vi "CRYAPI DOCKING LIB.vi"(6 "sData":string, 8 "tDFrame":T2, 9 "tSFrame":T2, 10 "nData":i32=2, 11 "sAction":string) -> (0 "nData_Out":i32=2, 1 "sData_Out":string, 3 "tFrame_Out":T2)   [LabVIEW 2013]
uses:
  <vilib>/Utility/miscctls.llb/LVRectTypeDef.ctl
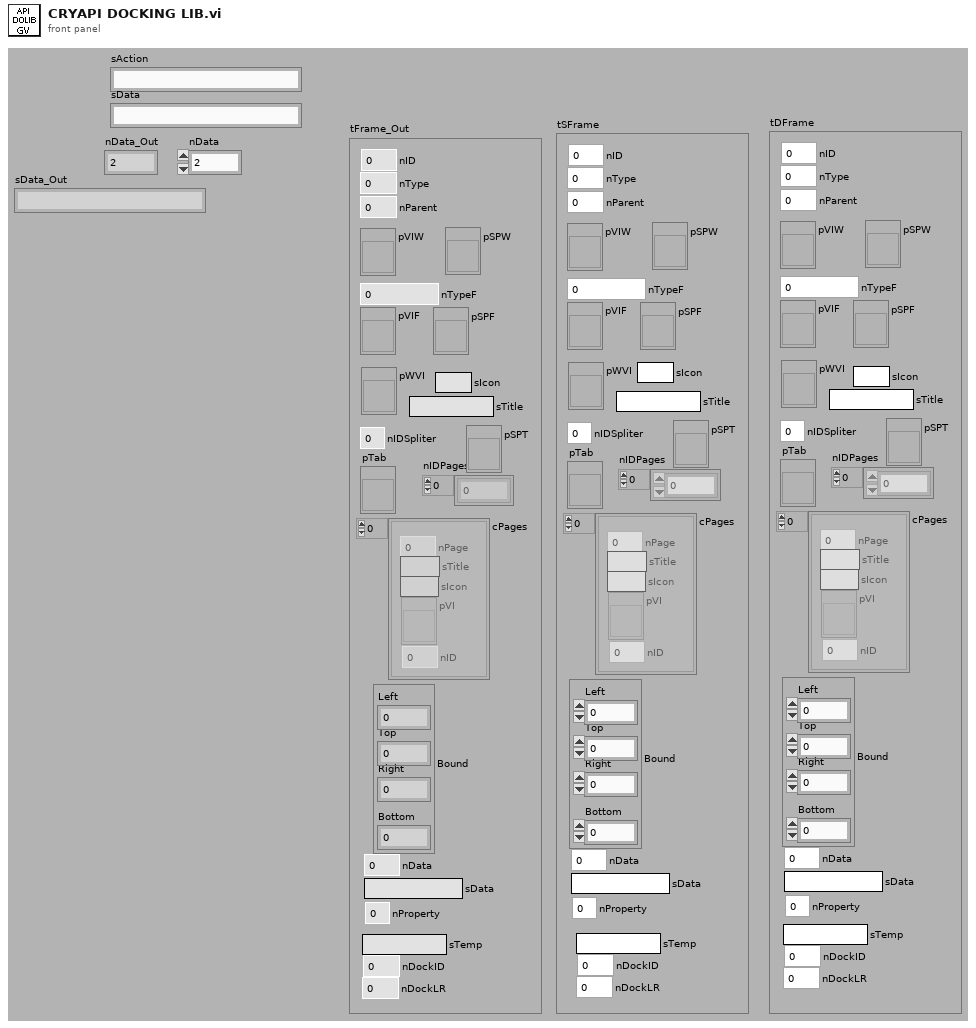
[diagram p1: front panel]
types:
  T1 = typedef "LVRectTypeDef.ctl" = cluster{"Left":i16, "Top":i16, "Right":i16, "Bottom":i16}
  T2 = cluster{"nType":i32, "nParent":i32, "pVIW":refnum<vi>, "pSPW":refnum<vi>, "nTypeF":i32, "pVIF":refnum<vi>, "pSPF":refnum<vi>, "nIDSpliter":i32, "nProperty":i32, "Bound":T1, "nID":i32, "nData":i32, "sData":string, "pWVI":refnum<vi>, "sTitle":string, "cPages":cluster{"nPage":i32, "sTitle":string, "sIcon":string, "pVI":refnum<vi>, "nID":i32}[], "pTab":refnum<vi>, "nIDPages":i32[], "pSPT":refnum<vi>, "sTemp":string, "nDockID":i32, "nDockLR":i32, "sIcon":string}
  T3 = cluster{"nPage":i32, "sTitle":string, "sIcon":string, "pVI":refnum<vi>, "nID":i32}[]
  T4 = cluster{"nType":i32, "nTypeP":i32, "pVI":refnum<vi>, "pSpliter":refnum<vi>, "pSPL":refnum<vi>, "pVIL":refnum<vi>, "pSPR":refnum<vi>, "pVIR":refnum<vi>, "nIDTL":i32, "nIDL":i32, "nIDTR":i32, "nIDR":i32, "nID":i32, "nIDParent":i32, "nData":i32, "sData":string}
  T5 = cluster{"pSP":refnum<vi>, "pVI":refnum<vi>, "nIDT":i32, "nID":i32, "nLR":i32}
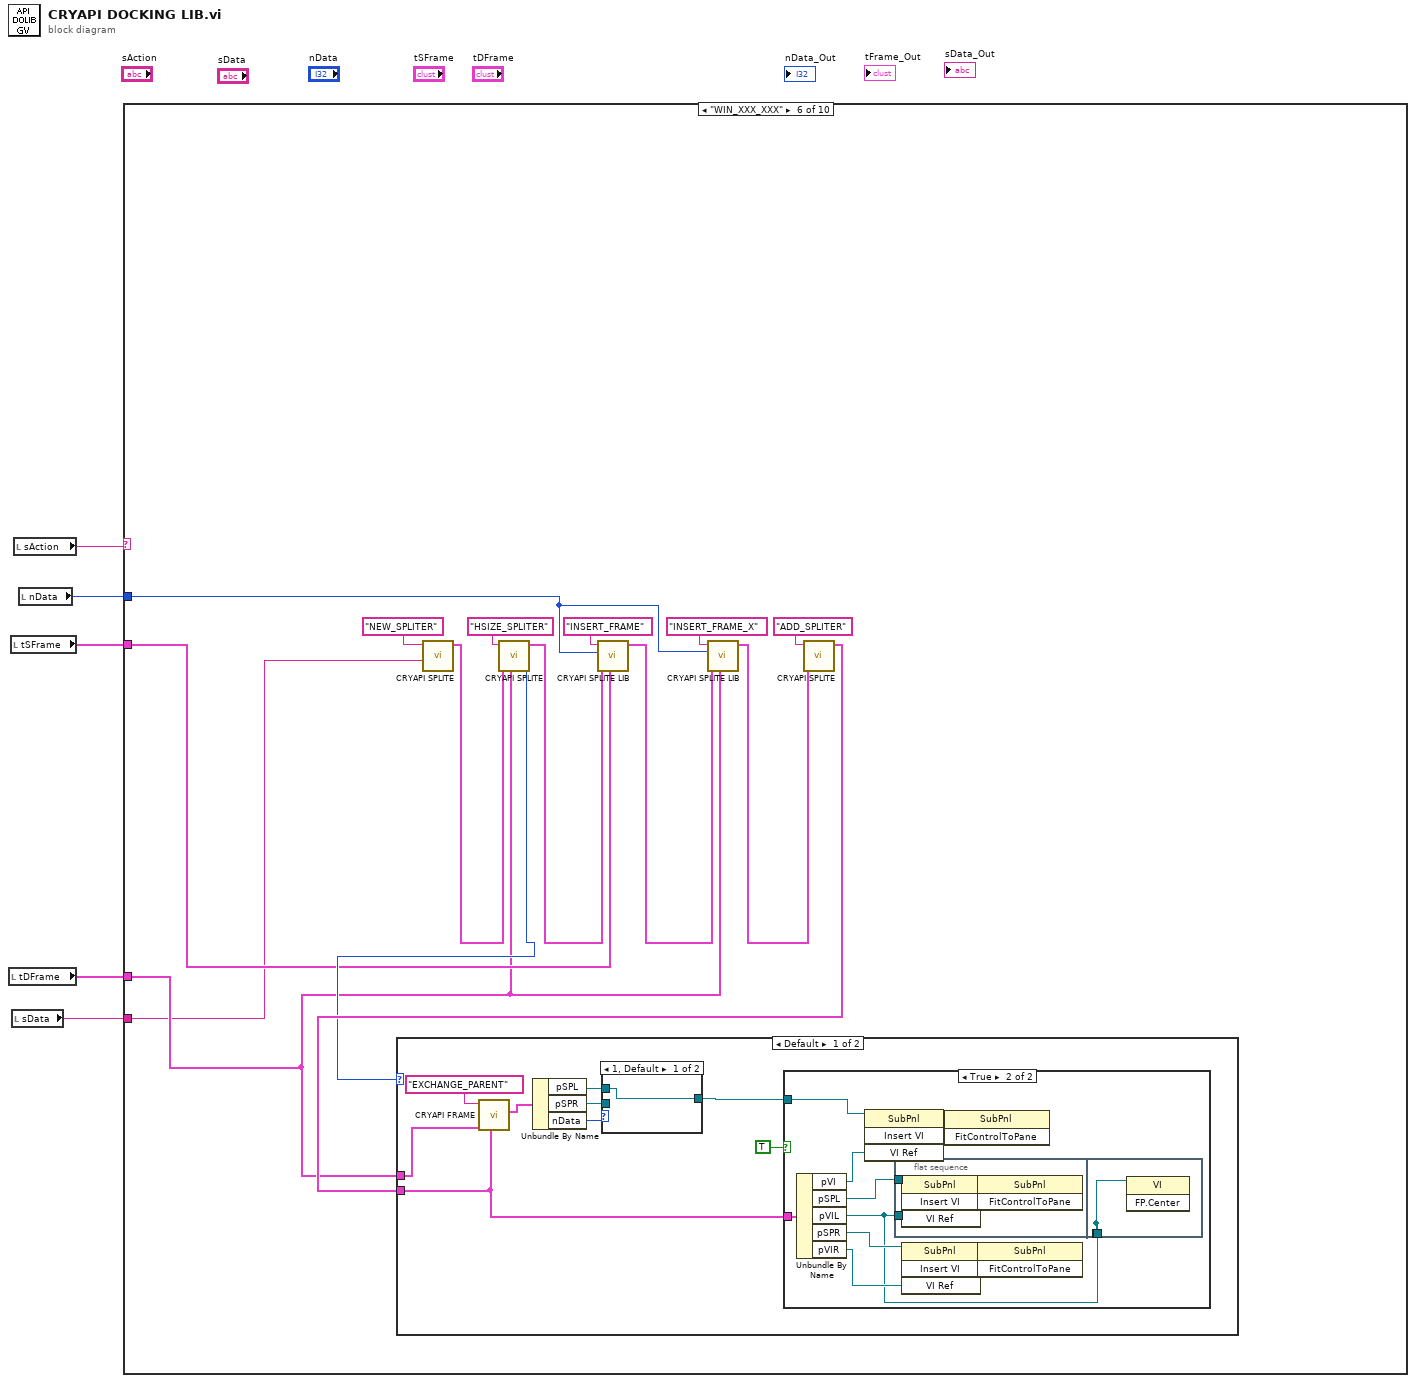
[diagram p0: block diagram]
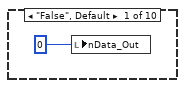
[diagram p2: hidden frame]
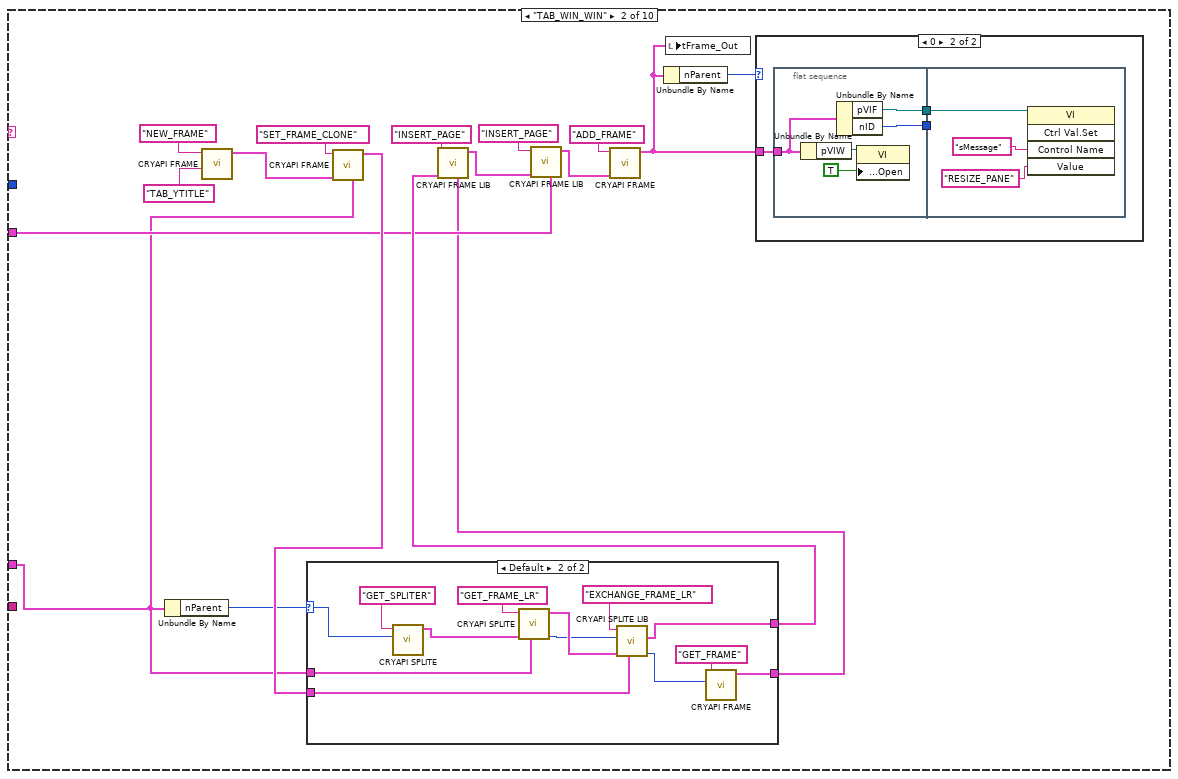
[diagram p3: hidden frame]
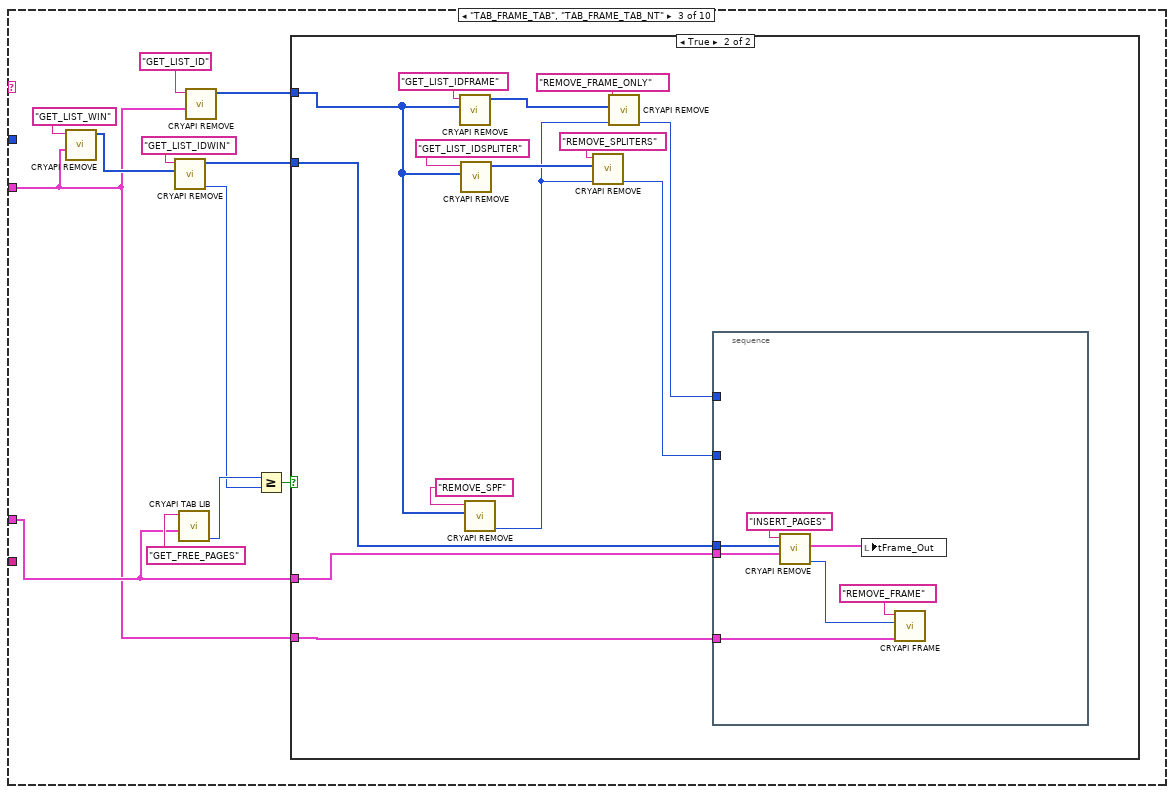
[diagram p6: hidden frame]
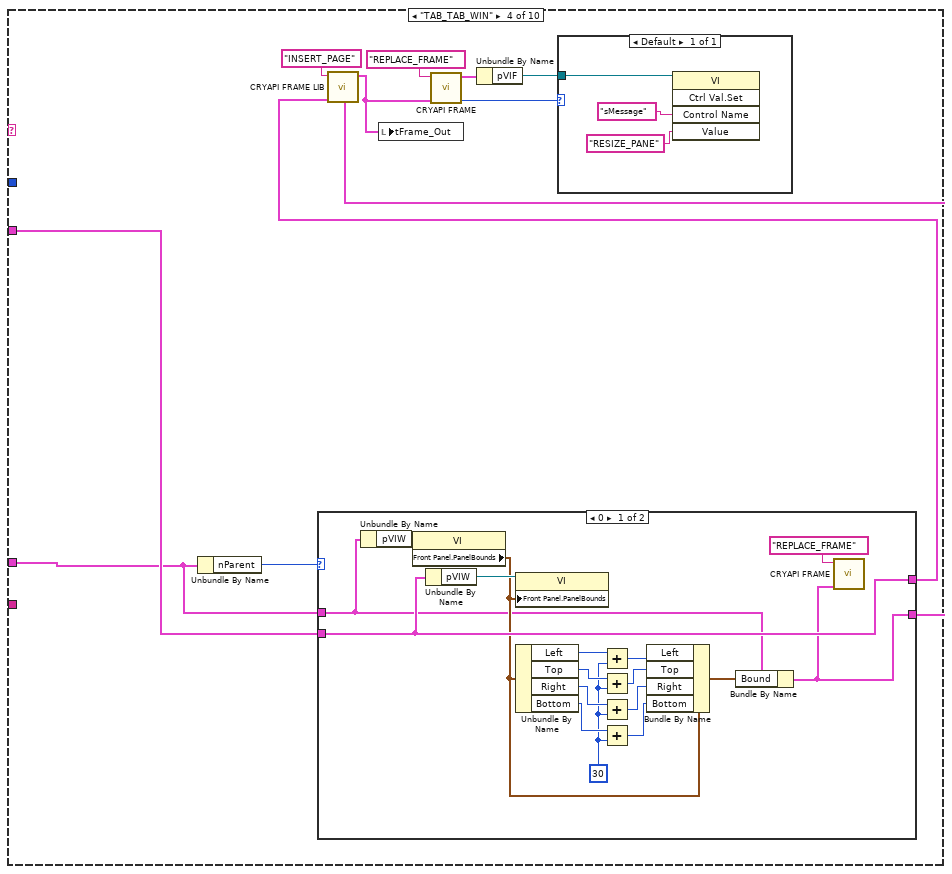
[diagram p8: hidden frame]
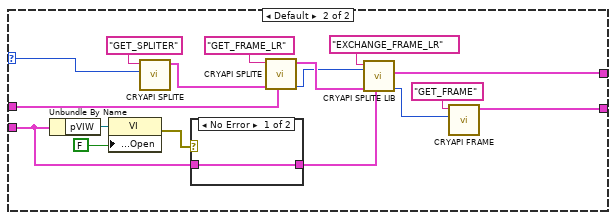
[diagram p9: hidden frame]
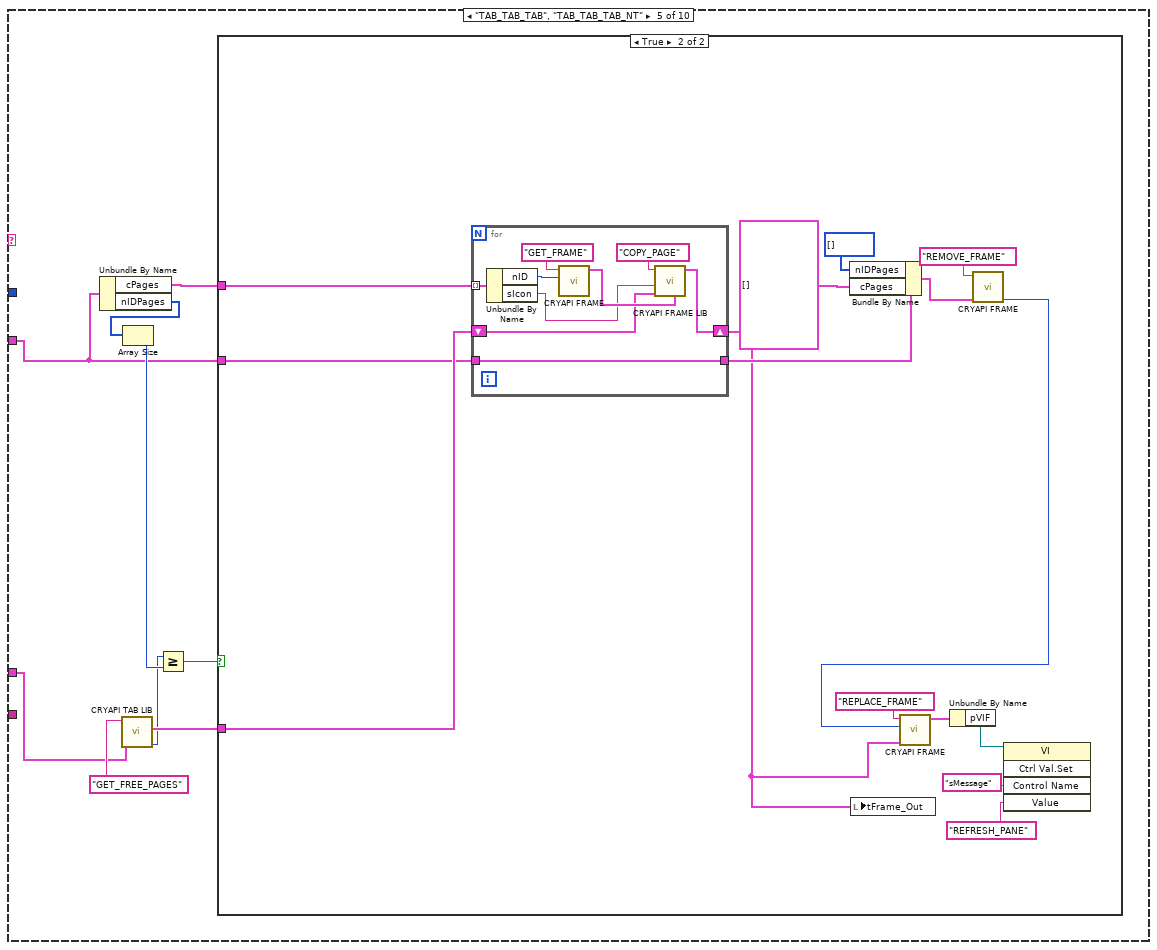
[diagram p11: hidden frame]
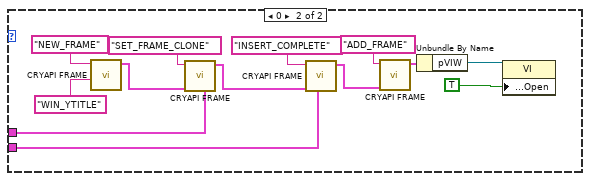
[diagram p15: hidden frame]
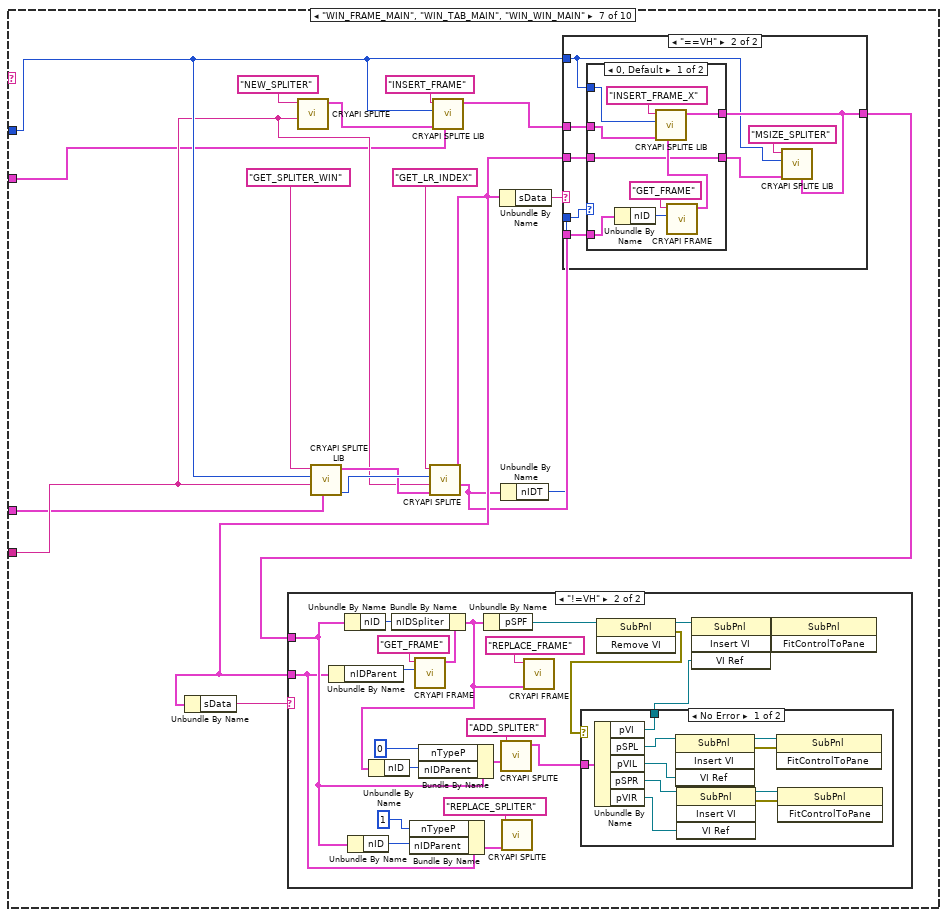
[diagram p16: hidden frame]
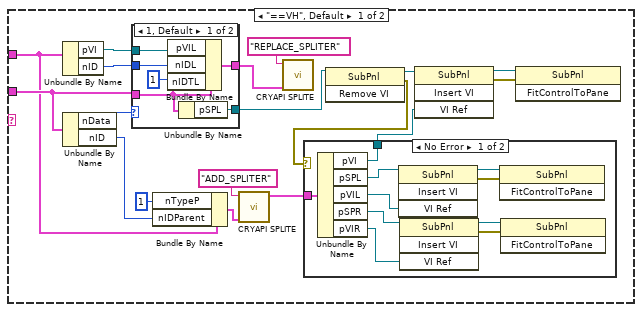
[diagram p17: hidden frame]
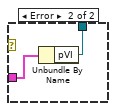
[diagram p18: hidden frame]
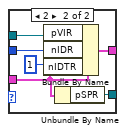
[diagram p19: hidden frame]
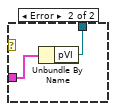
[diagram p20: hidden frame]
diagram:
  n1 = local read "tDFrame"() -> (w2:T2)
  n2 = local read "tSFrame"() -> (w3:T2)
  n3 = local read "sData"() -> (w1:string)
  n4 = local read "sAction"() -> (w5:string)
  n5 = local read "nData"() -> (w4:i32)
  n6 = case shown="\"WIN_XXX_XXX\"" w5 {
    selector: w5 -> [_ _ _ _ _ _ _ _ _ w510]
    tunnel: w4 -> [_ _ _ _ _ w167 w224 w351 w468 w512]
    tunnel: w3 -> [_ w10 w50 w85 w133 w169 w222 _ _ w509]
    tunnel: w2 -> [_ w9 w55 w84 w134 w168 w221 _ _ _]
    tunnel: w1 -> [_ _ _ _ _ w166 w223 w348 _ _]
    frame "False", Default {
      n7 = local write "nData_Out"(0 ("nData_Out")) -> ()
    }
    frame "TAB_WIN_WIN" {
      n8 = Unbundle By Name(w9) -> ("nParent"=w20:i32)
      n9 = call "CRYAPI FRAME.vi"("sData"="TAB_YTITLE", "sAction"="NEW_FRAME") -> ("tFrame_Out"=w11:T2)  [unwired: 4 in, 5 out]
      n10 = call "CRYAPI FRAME.vi"("tFrame_In"=w9, "tFrame"=w11, "sAction"="SET_FRAME_CLONE") -> ("tFrame_Out"=w21:T2)  [unwired: 3 in, 5 out]
      n11 = case shown="Default" w20 {
        selector: w20 -> [_ w40]
        tunnel: w21 -> [w36 w42]
        tunnel: [w36 w41] -> w22
        tunnel: w9 -> [w35 w47]
        tunnel: [w35 w37] -> w7
        frame 0 {
        }
        frame Default {
          n12 = call "CRYAPI SPLITE.vi"("nData"=w40, "sAction"="GET_SPLITER") -> ("tSpliter_Out"=w46:T4)  [unwired: 4 in, 5 out]
          n13 = call "CRYAPI SPLITE.vi"("tFrame"=w47, "tSpliter"=w46, "sAction"="GET_FRAME_LR") -> ("nData_Out"=w44:i32, "tSpliter_Out"=w45:T4)  [unwired: 3 in, 4 out]
          n14 = call "CRYAPI SPLITE LIB.vi"("tFrame"=w42, "tSpliter"=w45, "nData"=w44, "sAction"="EXCHANGE_FRAME_LR") -> ("nData_Out"=w38:i32, "tFrame_Out"=w41:T2)  [unwired: 2 in, 4 out]
          n15 = call "CRYAPI FRAME.vi"("nData"=w38, "sAction"="GET_FRAME") -> ("tFrame_Out"=w37:T2)  [unwired: 4 in, 5 out]
        }
      }
      n16 = call "CRYAPI FRAME LIB.vi"("tFrame_In"=w7, "tFrame"=w22, "sAction"="INSERT_PAGE") -> ("tFrame_Out"=w17:T2)  [unwired: 3 in, 5 out]
      n17 = call "CRYAPI FRAME LIB.vi"("tFrame_In"=w10, "tFrame"=w17, "sAction"="INSERT_PAGE") -> ("tFrame_Out"=w18:T2)  [unwired: 3 in, 5 out]
      n18 = call "CRYAPI FRAME.vi"("tFrame"=w18, "sAction"="ADD_FRAME") -> ("tFrame_Out"=w8:T2)  [unwired: 4 in, 5 out]
      n19 = Unbundle By Name(w8) -> ("nParent"=w23:i32)
      n20 = local write "tFrame_Out"(w8) -> ()
      n21 = case shown="0" w23 {
        tunnel: w8 -> [_ w26]
        frame Default {
        }
        frame 0 {
          n22 = flat-sequence {
            tunnel: w26 -> [w29]
            tunnel: [w28] -> w25
            tunnel: [w27] -> w24
            tunnel: w24 -> [_]
            tunnel: w25 -> [w32]
            frame #0 {
              n23 = Unbundle By Name(w29) -> ("pVIW"=w30:refnum<vi>)
              n24 = Unbundle By Name(w29) -> ("pVIF"=w28:refnum<vi>, "nID"=w27:i32)
              n25 = property class="VI"(reference=w30, "Front Panel.Open"=TRUE ("Front Panel Window:Open")) -> ()  [unwired: 1 in, 2 out]
            }
            frame #1 {
              n26 = invoke class="VI" method="Ctrl Val.Set"(reference=w32, "Control Name"="sMessage", "Value"="RESIZE_PANE" ("Control Name")) -> ()  [unwired: 2 in, 5 out]
            }
          }
        }
      }
    }
    frame "TAB_FRAME_TAB", "TAB_FRAME_TAB_NT" {
      n27 = call "CRYAPI REMOVE.vi"("tFrame"=w50, "sAction"="GET_LIST_WIN") -> ("List_ID_Out"=w52:i32[])  [unwired: 3 in, 6 out]
      n28 = call "CRYAPI REMOVE.vi"("List_ID"=w52, "sAction"="GET_LIST_IDWIN") -> ("nData_Out"=w53:i32, "List_ID_Out"=w51:i32[])  [unwired: 3 in, 5 out]
      n29 = call "CRYAPI TAB LIB.vi"("tFrame"=w55, "sAction"="GET_FREE_PAGES") -> ("nData_Out"=w58:i32)  [unwired: 2 in, 7 out]
      n30 = call "CRYAPI REMOVE.vi"("tFrame"=w50, "sAction"="GET_LIST_ID") -> ("List_ID_Out"=w61:i32[])  [unwired: 3 in, 6 out]
      n31 = Greater Or Equal?(x=w58, y=w53) -> (x >= y?=w60:bool)
      n32 = case shown="True" w60 {
        tunnel: w61 -> [_ w69]
        tunnel: w51 -> [_ w68]
        tunnel: w50 -> [_ w67]
        tunnel: w55 -> [_ w66]
        frame False {
        }
        frame True {
          n33 = call "CRYAPI REMOVE.vi"("List_ID"=w69, "sAction"="GET_LIST_IDFRAME") -> ("List_ID_Out"=w65:i32[])  [unwired: 3 in, 6 out]
          n34 = call "CRYAPI REMOVE.vi"("List_ID"=w69, "sAction"="GET_LIST_IDSPLITER") -> ("List_ID_Out"=w72:i32[])  [unwired: 3 in, 6 out]
          n35 = call "CRYAPI REMOVE.vi"("List_ID"=w69, "sAction"="REMOVE_SPF") -> ("nData_Out"=w64:i32)  [unwired: 3 in, 6 out]
          n36 = call "CRYAPI REMOVE.vi"("nData"=w64, "List_ID"=w72, "sAction"="REMOVE_SPLITERS") -> ("nData_Out"=w63:i32)  [unwired: 2 in, 6 out]
          n37 = call "CRYAPI REMOVE.vi"("nData"=w64, "List_ID"=w65, "sAction"="REMOVE_FRAME_ONLY") -> ("nData_Out"=w62:i32)  [unwired: 2 in, 6 out]
          n38 = stacked-sequence {
            tunnel: w68 -> [w81]
            tunnel: w67 -> [w79]
            tunnel: w66 -> [w77]
            tunnel: w63 -> [_]
            tunnel: w62 -> [_]
            frame #0 {
              n39 = call "CRYAPI REMOVE.vi"("tFrame"=w77, "List_ID"=w81, "sAction"="INSERT_PAGES") -> ("nData_Out"=w78:i32, "tFrame_Out"=w76:T2)  [unwired: 2 in, 5 out]
              n40 = local write "tFrame_Out"(w76) -> ()
              n41 = call "CRYAPI FRAME.vi"("tFrame"=w79, "nData"=w78, "sAction"="REMOVE_FRAME") -> ()  [unwired: 3 in, 6 out]
            }
          }
        }
      }
    }
    frame "TAB_TAB_WIN" {
      n42 = Unbundle By Name(w84) -> ("nParent"=w90:i32)
      n43 = case shown="0" w90 {
        selector: w90 -> [_ w119]
        tunnel: w85 -> [w108 w115]
        tunnel: [w108 w120] -> w91
        tunnel: w84 -> [w97 w125]
        tunnel: [w94 w111] -> w92
        frame 0 {
          w98 = 30
          n44 = Unbundle By Name(w97) -> ("pVIW"=w110:refnum<vi>)
          n45 = property class="VI"(reference=w110) -> ("Front Panel.PanelBounds"=w107:T1)  [unwired: 1 in, 2 out]
          n46 = Unbundle By Name(w108) -> ("pVIW"=w109:refnum<vi>)
          n47 = property class="VI"(reference=w109, "Front Panel.PanelBounds"=w107) -> ()  [unwired: 1 in, 2 out]
          n48 = Unbundle By Name(w107) -> ("Left"=w102:i16, "Top"=w101:i16, "Right"=w100:i16, "Bottom"=w99:i16)
          n49 = Add(x=w102, y=w98) -> (x+y=w106:i32)
          n50 = Add(x=w101, y=w98) -> (x+y=w105:i32)
          n51 = Add(x=w100, y=w98) -> (x+y=w104:i32)
          n52 = Add(x=w99, y=w98) -> (x+y=w103:i32)
          n53 = Bundle By Name(cluster=w107, "Left"=w106, "Top"=w105, "Right"=w104, "Bottom"=w103) -> (w96:T1)
          n54 = Bundle By Name(cluster=w97, "Bound"=w96) -> (w94:T2)
          n55 = call "CRYAPI FRAME.vi"("tFrame"=w94, "sAction"="REPLACE_FRAME") -> ()  [unwired: 4 in, 6 out]
        }
        frame Default {
          n56 = Unbundle By Name(w115) -> ("pVIW"=w118:refnum<vi>)
          n57 = property class="VI"(reference=w118, "Front Panel.Open"=FALSE ("Front Panel Window:Open")) -> (error out=w116:errorcluster)  [unwired: 1 in, 1 out]
          n58 = call "CRYAPI SPLITE.vi"("nData"=w119, "sAction"="GET_SPLITER") -> ("tSpliter_Out"=w124:T4)  [unwired: 4 in, 5 out]
          n59 = case shown="No Error" w116 {
            tunnel: w115 -> [w128 w129]
            tunnel: [w128 w129] -> w114
            frame No Error {
            }
            frame Error {
            }
          }
          n60 = call "CRYAPI SPLITE.vi"("tFrame"=w125, "tSpliter"=w124, "sAction"="GET_FRAME_LR") -> ("nData_Out"=w122:i32, "tSpliter_Out"=w123:T4)  [unwired: 3 in, 4 out]
          n61 = call "CRYAPI SPLITE LIB.vi"("tFrame"=w114, "tSpliter"=w123, "nData"=w122, "sAction"="EXCHANGE_FRAME_LR") -> ("nData_Out"=w112:i32, "tFrame_Out"=w120:T2)  [unwired: 2 in, 4 out]
          n62 = call "CRYAPI FRAME.vi"("nData"=w112, "sAction"="GET_FRAME") -> ("tFrame_Out"=w111:T2)  [unwired: 4 in, 5 out]
        }
      }
      n63 = call "CRYAPI FRAME LIB.vi"("tFrame_In"=w92, "tFrame"=w91, "sAction"="INSERT_PAGE") -> ("tFrame_Out"=w83:T2)  [unwired: 3 in, 5 out]
      n64 = local write "tFrame_Out"(w83) -> ()
      n65 = call "CRYAPI FRAME.vi"("tFrame"=w83, "sAction"="REPLACE_FRAME") -> ("nData_Out"=w93:i32, "tFrame_Out"=w88:T2)  [unwired: 4 in, 4 out]
      n66 = Unbundle By Name(w88) -> ("pVIF"=w89:refnum<vi>)
      n67 = case shown="Default" w93 {
        tunnel: w89 -> [w132]
        frame Default {
          n68 = invoke class="VI" method="Ctrl Val.Set"(reference=w132, "Control Name"="sMessage", "Value"="RESIZE_PANE" ("Control Name")) -> ()  [unwired: 2 in, 5 out]
        }
      }
    }
    frame "TAB_TAB_TAB", "TAB_TAB_TAB_NT" {
      n69 = Unbundle By Name(w133) -> ("cPages"=w141:T3, "nIDPages"=w139:i32[])
      n70 = call "CRYAPI TAB LIB.vi"("tFrame"=w134, "sAction"="GET_FREE_PAGES") -> ("nData_Out"=w136:i32, "tFrame_Out"=w140:T2)  [unwired: 2 in, 6 out]
      n71 = Array Size(array=w139) -> (size(s)=w137:i32)
      n72 = Greater Or Equal?(x=w136, y=w137) -> (x >= y?=w138:bool)
      n73 = case shown="True" w138 {
        tunnel: w140 -> [_ w156]
        tunnel: w133 -> [_ w142]
        tunnel: w141 -> [_ w152]
        frame False {
        }
        frame True {
          n74 = for {
            shift-right: [w162] -> w148
            shift-left: w156 -> [w161]
            tunnel: w142 -> [w160]
            tunnel: [w160] -> w155
            tunnel: w152 -> [w159] mode=indexing
            n75 = Unbundle By Name(w159) -> ("nID"=w157:i32, "sIcon"=w158:string)
            n76 = call "CRYAPI FRAME.vi"("nData"=w157, "sAction"="GET_FRAME") -> ("tFrame_Out"=w163:T2)  [unwired: 4 in, 5 out]
            n77 = call "CRYAPI FRAME LIB.vi"("tFrame_In"=w163, "tFrame"=w161, "sData"=w158, "sAction"="COPY_PAGE") -> ("tFrame_Out"=w162:T2)  [unwired: 2 in, 5 out]
          }
          n78 = Bundle By Name(cluster=w155, "nIDPages"=i32[] [], "cPages"=T3 []) -> (w149:T2)
          n79 = local write "tFrame_Out"(w148) -> ()
          n80 = call "CRYAPI FRAME.vi"("tFrame"=w149, "sAction"="REMOVE_FRAME") -> ("nData_Out"=w143:i32)  [unwired: 4 in, 5 out]
          n81 = call "CRYAPI FRAME.vi"("tFrame"=w148, "nData"=w143, "sAction"="REPLACE_FRAME") -> ("tFrame_Out"=w150:T2)  [unwired: 3 in, 5 out]
          n82 = Unbundle By Name(w150) -> ("pVIF"=w147:refnum<vi>)
          n83 = invoke class="VI" method="Ctrl Val.Set"(reference=w147, "Control Name"="sMessage", "Value"="REFRESH_PANE" ("sAction")) -> ()  [unwired: 2 in, 5 out]
        }
      }
    }
    frame "WIN_XXX_XXX" {
      n84 = call "CRYAPI SPLITE.vi"("sData"=w166, "sAction"="NEW_SPLITER") -> ("tSpliter_Out"=w170:T4)  [unwired: 4 in, 5 out]
      n85 = call "CRYAPI SPLITE.vi"("tFrame"=w168, "tSpliter"=w170, "sAction"="HSIZE_SPLITER") -> ("nData_Out"=w176:i32, "tSpliter_Out"=w177:T4)  [unwired: 3 in, 4 out]
      n86 = call "CRYAPI SPLITE LIB.vi"("tFrame"=w169, "tSpliter"=w177, "nData"=w167, "sAction"="INSERT_FRAME") -> ("tSpliter_Out"=w175:T4)  [unwired: 2 in, 5 out]
      n87 = call "CRYAPI SPLITE LIB.vi"("tFrame"=w168, "tSpliter"=w175, "nData"=w167, "sAction"="INSERT_FRAME_X") -> ("tSpliter_Out"=w179:T4)  [unwired: 2 in, 5 out]
      n88 = call "CRYAPI SPLITE.vi"("tSpliter"=w179, "sAction"="ADD_SPLITER") -> ("tSpliter_Out"=w180:T4)  [unwired: 4 in, 5 out]
      n89 = case shown="Default" w176 {
        tunnel: w168 -> [w188 w216]
        tunnel: w180 -> [w187 w208]
        frame Default {
          n90 = call "CRYAPI FRAME.vi"("tSpliter"=w187, "tFrame"=w188, "sAction"="EXCHANGE_PARENT") -> ("tSpliter_Out"=w185:T4)  [unwired: 3 in, 5 out]
          n91 = Unbundle By Name(w185) -> ("pSPL"=w184:refnum<vi>, "pSPR"=w183:refnum<vi>, "nData"=w186:i32)
          n92 = case shown="1, Default" w186 {
            tunnel: w184 -> [w206 _]
            tunnel: w183 -> [_ w207]
            tunnel: [w206 w207] -> w182
            frame 1, Default {
            }
            frame 2 {
            }
          }
          n93 = case shown="True" TRUE {
            tunnel: w187 -> [_ w200]
            tunnel: w182 -> [_ w199]
            frame False {
            }
            frame True {
              n94 = Unbundle By Name(w200) -> ("pVI"=w196:refnum<vi>, "pSPL"=w191:refnum<vi>, "pVIL"=w190:refnum<vi>, "pSPR"=w194:refnum<vi>, "pVIR"=w195:refnum<vi>)
              n95 = invoke class="SubPnl" method="Insert VI"(reference=w199, "VI Ref"=w196) -> (reference out=w198:refnum<vi>, error out=w197:errorcluster)  [unwired: 2 in, 2 out]
              n96 = flat-sequence {
                tunnel: w190 -> [w203]
                tunnel: w191 -> [w202]
                tunnel: [w205] -> _
                tunnel: w190 -> [w205]
                frame #0 {
                  n97 = invoke class="SubPnl" method="Insert VI"(reference=w202, "VI Ref"=w203) -> (reference out=w201:refnum<vi>, error out=w204:errorcluster)  [unwired: 2 in, 2 out]
                  n98 = invoke class="SubPnl" method="FitControlToPane"(reference=w201, error in=w204) -> ()  [unwired: 1 in, 3 out]
                }
                frame #1 {
                  n99 = invoke class="VI" method="FP.Center"(reference=w205) -> ()  [unwired: 2 in, 3 out]
                }
              }
              n100 = invoke class="SubPnl" method="Insert VI"(reference=w194, "VI Ref"=w195) -> (reference out=w193:refnum<vi>, error out=w192:errorcluster)  [unwired: 2 in, 2 out]
              n101 = invoke class="SubPnl" method="FitControlToPane"(reference=w198, error in=w197) -> ()  [unwired: 1 in, 3 out]
              n102 = invoke class="SubPnl" method="FitControlToPane"(reference=w193, error in=w192) -> ()  [unwired: 1 in, 3 out]
            }
          }
        }
        frame 0 {
          n103 = call "CRYAPI FRAME.vi"("sData"="WIN_YTITLE", "sAction"="NEW_FRAME") -> ("tFrame_Out"=w220:T2)  [unwired: 4 in, 5 out]
          n104 = call "CRYAPI FRAME.vi"("tFrame_In"=w216, "tFrame"=w220, "sAction"="SET_FRAME_CLONE") -> ("tFrame_Out"=w209:T2)  [unwired: 3 in, 5 out]
          n105 = call "CRYAPI FRAME.vi"("tSpliter"=w208, "tFrame"=w209, "sAction"="INSERT_COMPLETE") -> ("tFrame_Out"=w212:T2)  [unwired: 3 in, 5 out]
          n106 = call "CRYAPI FRAME.vi"("tFrame"=w212, "sAction"="ADD_FRAME") -> ("tFrame_Out"=w214:T2)  [unwired: 4 in, 5 out]
          n107 = Unbundle By Name(w214) -> ("pVIW"=w215:refnum<vi>)
          n108 = property class="VI"(reference=w215, "Front Panel.Open"=TRUE ("Front Panel Window:Open")) -> ()  [unwired: 1 in, 2 out]
        }
      }
    }
    frame "WIN_FRAME_MAIN", "WIN_TAB_MAIN", "WIN_WIN_MAIN" {
      n109 = call "CRYAPI SPLITE.vi"("sData"=w223, "sAction"="NEW_SPLITER") -> ("tSpliter_Out"=w232:T4)  [unwired: 4 in, 5 out]
      n110 = call "CRYAPI SPLITE LIB.vi"("tFrame"=w221, "sData"=w223, "nData"=w224, "sAction"="GET_SPLITER_WIN") -> ("nData_Out"=w238:i32, "tSpliter_Out"=w231:T4)  [unwired: 2 in, 4 out]
      n111 = call "CRYAPI SPLITE.vi"("tSpliter"=w231, "sData"=w223, "nData"=w238, "sAction"="GET_LR_INDEX") -> ("tLR_Out"=w233:T5, "tSpliter_Out"=w237:T4)  [unwired: 2 in, 4 out]
      n112 = Unbundle By Name(w237) -> ("sData"=w236:string)
      n113 = call "CRYAPI SPLITE LIB.vi"("tFrame"=w222, "tSpliter"=w232, "nData"=w224, "sAction"="INSERT_FRAME") -> ("tSpliter_Out"=w228:T4)  [unwired: 2 in, 5 out]
      n114 = Unbundle By Name(w237) -> ("sData"=w235:string)
      n115 = Unbundle By Name(w233) -> ("nIDT"=w230:i32)
      n116 = case shown="\"==VH\"" w235 {
        tunnel: w228 -> [w320 w329]
        tunnel: [w316 w323] -> w234
        tunnel: w224 -> [w317 w322]
        tunnel: w230 -> [_ w328]
        tunnel: w233 -> [_ w327]
        tunnel: w237 -> [w318 w325]
        frame "!=VH", Default {
          n117 = call "CRYAPI SPLITE LIB.vi"("tSpliter_In"=w318, "tSpliter"=w320, "nData"=w317, "sAction"="INSERT_SPLITER_X") -> ("tSpliter_Out"=w316:T4)  [unwired: 2 in, 5 out]
          n118 = call "CRYAPI SPLITE.vi"("tSpliter_In"=w316, "tSpliter"=w318, "nData"=w317, "sAction"="TSIZE_SPLITER") -> ()  [unwired: 2 in, 6 out]
        }
        frame "==VH" {
          n119 = case shown="0, Default" w328 {
            tunnel: w329 -> [w333 w345]
            tunnel: [w334 w346] -> w323
            tunnel: w322 -> [w332 w344]
            tunnel: w327 -> [w331 w343]
            tunnel: [w330 w339] -> w324
            tunnel: w325 -> [w330 w339]
            frame 0, Default {
              n120 = Unbundle By Name(w331) -> ("nID"=w337:i32)
              n121 = call "CRYAPI FRAME.vi"("nData"=w337, "sAction"="GET_FRAME") -> ("tFrame_Out"=w335:T2)  [unwired: 4 in, 5 out]
              n122 = call "CRYAPI SPLITE LIB.vi"("tFrame"=w335, "tSpliter"=w333, "nData"=w332, "sAction"="INSERT_FRAME_X") -> ("tSpliter_Out"=w334:T4)  [unwired: 2 in, 5 out]
            }
            frame 1 {
              n123 = Unbundle By Name(w343) -> ("nID"=w342:i32)
              n124 = call "CRYAPI SPLITE.vi"("nData"=w342, "sAction"="GET_SPLITER") -> ("tSpliter_Out"=w340:T4)  [unwired: 4 in, 5 out]
              n125 = call "CRYAPI SPLITE LIB.vi"("tSpliter_In"=w340, "tSpliter"=w345, "nData"=w344, "sAction"="INSERT_SPLITER_X") -> ("tSpliter_Out"=w346:T4)  [unwired: 2 in, 5 out]
            }
          }
          n126 = call "CRYAPI SPLITE LIB.vi"("tSpliter_In"=w323, "tSpliter"=w324, "nData"=w322, "sAction"="MSIZE_SPLITER") -> ()  [unwired: 2 in, 6 out]
        }
      }
      n127 = case shown="\"!=VH\"" w236 {
        tunnel: w234 -> [w251 w283]
        tunnel: w237 -> [w253 w281]
        frame "==VH", Default {
          n128 = Unbundle By Name(w251) -> ("pVI"=w255:refnum<vi>, "nID"=w254:i32)
          n129 = Unbundle By Name(w253) -> ("nData"=w256:i32, "nID"=w250:i32)
          n130 = case shown="1, Default" w256 {
            tunnel: [w274 w280] -> w239
            tunnel: [w270 w276] -> w240
            tunnel: w255 -> [w272 w278]
            tunnel: w254 -> [w271 w277]
            tunnel: w253 -> [w269 w275]
            frame 1, Default {
              n131 = Bundle By Name(cluster=w269, "pVIL"=w272, "nIDL"=w271, "nIDTL"=1) -> (w270:T4)
              n132 = Unbundle By Name(w269) -> ("pSPL"=w274:refnum<vi>)
            }
            frame 2 {
              n133 = Bundle By Name(cluster=w275, "pVIR"=w278, "nIDR"=w277, "nIDTR"=1 ("nIDTL")) -> (w276:T4)
              n134 = Unbundle By Name(w275) -> ("pSPR"=w280:refnum<vi>)
            }
          }
          n135 = Bundle By Name(cluster=w251, "nTypeP"=1, "nIDParent"=w250) -> (w248:T4)
          n136 = call "CRYAPI SPLITE.vi"("tSpliter"=w248, "sAction"="ADD_SPLITER") -> ("tSpliter_Out"=w242:T4)  [unwired: 4 in, 5 out]
          n137 = call "CRYAPI SPLITE.vi"("tSpliter"=w240, "sAction"="REPLACE_SPLITER") -> ()  [unwired: 4 in, 6 out]
          n138 = invoke class="SubPnl" method="Remove VI"(reference=w239) -> (reference out=w243:refnum<vi>, error out=w246:errorcluster)  [unwired: 2 in, 1 out]
          n139 = case shown="No Error" w246 {
            tunnel: w242 -> [w258 w268]
            tunnel: [w257 w267] -> w247
            frame No Error {
              n140 = Unbundle By Name(w258) -> ("pVI"=w257:refnum<vi>, "pSPL"=w265:refnum<vi>, "pVIL"=w264:refnum<vi>, "pSPR"=w260:refnum<vi>, "pVIR"=w259:refnum<vi>)
              n141 = invoke class="SubPnl" method="Insert VI"(reference=w265, "VI Ref"=w264) -> (reference out=w266:refnum<vi>, error out=w263:errorcluster)  [unwired: 2 in, 2 out]
              n142 = invoke class="SubPnl" method="Insert VI"(reference=w260, "VI Ref"=w259) -> (reference out=w261:refnum<vi>, error out=w262:errorcluster)  [unwired: 2 in, 2 out]
              n143 = invoke class="SubPnl" method="FitControlToPane"(reference=w266, error in=w263) -> ()  [unwired: 1 in, 3 out]
              n144 = invoke class="SubPnl" method="FitControlToPane"(reference=w261, error in=w262) -> ()  [unwired: 1 in, 3 out]
            }
            frame Error {
              n145 = Unbundle By Name(w268) -> ("pVI"=w267:refnum<vi>)
            }
          }
          n146 = invoke class="SubPnl" method="Insert VI"(reference=w243, "VI Ref"=w247) -> (reference out=w245:refnum<vi>, error out=w244:errorcluster)  [unwired: 2 in, 2 out]
          n147 = invoke class="SubPnl" method="FitControlToPane"(reference=w245, error in=w244) -> ()  [unwired: 1 in, 3 out]
        }
        frame "!=VH" {
          n148 = Unbundle By Name(w281) -> ("nIDParent"=w302:i32)
          n149 = Unbundle By Name(w283) -> ("nID"=w300:i32)
          n150 = Unbundle By Name(w283) -> ("nID"=w284:i32)
          n151 = Bundle By Name(cluster=w281, "nTypeP"=1, "nIDParent"=w284) -> (w285:T4)
          n152 = call "CRYAPI FRAME.vi"("nData"=w302, "sAction"="GET_FRAME") -> ("tFrame_Out"=w301:T2)  [unwired: 4 in, 5 out]
          n153 = Bundle By Name(cluster=w301, "nIDSpliter"=w300) -> (w287:T2)
          n154 = Unbundle By Name(w287) -> ("nID"=w288:i32)
          n155 = Bundle By Name(cluster=w283, "nTypeP"=0, "nIDParent"=w288) -> (w298:T4)
          n156 = Unbundle By Name(w287) -> ("pSPF"=w292:refnum<vi>)
          n157 = call "CRYAPI SPLITE.vi"("tSpliter"=w298, "sAction"="ADD_SPLITER") -> ("tSpliter_Out"=w289:T4)  [unwired: 4 in, 5 out]
          n158 = call "CRYAPI SPLITE.vi"("tSpliter"=w285, "sAction"="REPLACE_SPLITER") -> ()  [unwired: 4 in, 6 out]
          n159 = call "CRYAPI FRAME.vi"("tFrame"=w287, "sAction"="REPLACE_FRAME") -> ()  [unwired: 4 in, 6 out]
          n160 = invoke class="SubPnl" method="Remove VI"(reference=w292) -> (reference out=w295:refnum<vi>, error out=w291:errorcluster)  [unwired: 2 in, 1 out]
          n161 = case shown="No Error" w291 {
            tunnel: w289 -> [w305 w315]
            tunnel: [w304 w314] -> w290
            frame No Error {
              n162 = Unbundle By Name(w305) -> ("pVI"=w304:refnum<vi>, "pSPL"=w312:refnum<vi>, "pVIL"=w311:refnum<vi>, "pSPR"=w307:refnum<vi>, "pVIR"=w306:refnum<vi>)
              n163 = invoke class="SubPnl" method="Insert VI"(reference=w312, "VI Ref"=w311) -> (reference out=w313:refnum<vi>, error out=w310:errorcluster)  [unwired: 2 in, 2 out]
              n164 = invoke class="SubPnl" method="Insert VI"(reference=w307, "VI Ref"=w306) -> (reference out=w308:refnum<vi>, error out=w309:errorcluster)  [unwired: 2 in, 2 out]
              n165 = invoke class="SubPnl" method="FitControlToPane"(reference=w313, error in=w310) -> ()  [unwired: 1 in, 3 out]
              n166 = invoke class="SubPnl" method="FitControlToPane"(reference=w308, error in=w309) -> ()  [unwired: 1 in, 3 out]
            }
            frame Error {
              n167 = Unbundle By Name(w315) -> ("pVI"=w314:refnum<vi>)
            }
          }
          n168 = invoke class="SubPnl" method="Insert VI"(reference=w295, "VI Ref"=w290) -> (reference out=w293:refnum<vi>, error out=w294:errorcluster)  [unwired: 2 in, 2 out]
          n169 = invoke class="SubPnl" method="FitControlToPane"(reference=w293, error in=w294) -> ()  [unwired: 1 in, 3 out]
        }
      }
    }
    frame "CHECK_PARENT" {
      # "Parent is 0:Error 1:MAIN 2:WIN_NT 3:TAB_NT 4:WIN 5:TAB"
      n170 = case shown="Default" w351 {
        selector: w351 -> [w353 w366]
        tunnel: [1 ("nData_Out") w357] -> w350
        tunnel: [w352 w358] -> w349
        tunnel: w348 -> [_ w361]
        frame 1 {
          n171 = call "CRYAPI FRAME.vi"("nData"=w353, "sAction"="GET_FRAME") -> ("tFrame_Out"=w352:T2)  [unwired: 4 in, 5 out]
        }
        frame Default {
          n172 = call "CRYAPI FRAME.vi"("nData"=w366, "sAction"="GET_FRAME") -> ("tFrame_Out"=w362:T2)  [unwired: 4 in, 5 out]
          n173 = Unbundle By Name(w362) -> ("nParent"=w365:i32, "nTypeF"=w364:i32, "nType"=w363:i32)
          n174 = case shown="1.." w365 {
            selector: w365 -> [_ w433 w450]
            tunnel: w364 -> [w414 _ w455]
            tunnel: w363 -> [w413 _ _]
            tunnel: w362 -> [w412 w425 w459]
            tunnel: w361 -> [_ _ w458]
            tunnel: [w412 w424 w451] -> w360
            tunnel: [w411 w429 w450] -> w359
            tunnel: [FALSE w428 TRUE] -> w356
            frame 0, Default {
              n175 = case shown="0, Default" w414 {
                tunnel: w413 -> [w416 w420]
                tunnel: [w415 w419] -> w411
                frame 0, Default {
                  n176 = case shown="Default" w416 {
                    tunnel: [2 4] -> w415
                    frame 0 {
                    }
                    frame Default {
                    }
                  }
                }
                frame 1 {
                  n177 = case shown="Default" w420 {
                    tunnel: [3 5] -> w419
                    frame 0 {
                    }
                    frame Default {
                    }
                  }
                }
              }
            }
            frame 1.. {
              n178 = call "CRYAPI FRAME.vi"("nData"=w433, "sAction"="GET_FRAME") -> ("tFrame_Out"=w426:T2)  [unwired: 4 in, 5 out]
              n179 = Unbundle By Name(w426) -> ("nTypeF"=w427:i32, "nType"=w432:i32, "nParent"=w423:i32)
              n180 = Less Than 0?(x=w423) -> (x < 0?=w431:bool)
              n181 = case shown="1" w427 {
                tunnel: w432 -> [w442 w446]
                tunnel: [w441 w445] -> w430
                frame 0, Default {
                  n182 = case shown="0" w442 {
                    tunnel: [2 4] -> w441
                    frame 0 {
                    }
                    frame Default {
                    }
                  }
                }
                frame 1 {
                  n183 = case shown="Default" w446 {
                    tunnel: [3 5] -> w445
                    frame 0 {
                    }
                    frame Default {
                    }
                  }
                }
              }
              n184 = case shown="False" w431 {
                selector: w431 -> [w437 w439]
                tunnel: w423 -> [_ w440]
                tunnel: [w438 w440] -> w429
                tunnel: [w437 w439] -> w428
                tunnel: w430 -> [w438 _]
                frame False {
                }
                frame True {
                }
              }
              n185 = case shown="1" w427 {
                tunnel: w426 -> [_ w436]
                tunnel: w425 -> [w435 _]
                tunnel: [w435 w436] -> w424
                frame 0, Default {
                }
                frame 1 {
                }
              }
            }
            frame ..-1 {
              n186 = Equal?(x=w458, y="DOCK_CENTER") -> (x = y?=w452:bool)
              n187 = Equal?(x=w455, y=1) -> (x = y?=w453:bool)
              n188 = And(x=w453, y=w452) -> (x .and. y?=w456:bool)
              n189 = case shown="False" w456 {
                tunnel: [w460 T2 {"nType"=0, "nParent"=0, "pVIW"=refnum, "pSPW"=refnum, "nTypeF"=0, "pVIF"=refnum, "pSPF"=refnum, "nIDSpliter"=0, "nProperty"=0, "Bound"={"Left"=0, "Top"=0, "Right"=0, "Bottom"=0}, "nID"=0, "nData"=0, "sData"="", "pWVI"=refnum, "sTitle"="", "cPages"=[], "pTab"=refnum, "nIDPages"=[], "pSPT"=refnum, "sTemp"="", "nDockID"=0, "nDockLR"=0, "sIcon"=""} ("tFrame_Out")] -> w451
                tunnel: w459 -> [w460 _]
                frame True {
                }
                frame False {
                }
              }
            }
          }
          n190 = case shown="True" w356 {
            tunnel: w360 -> [w369 w373]
            tunnel: w359 -> [w368 w372]
            tunnel: [w369 w371] -> w358
            tunnel: [w368 w370] -> w357
            frame False {
            }
            frame True {
              n191 = while {
                shift-right: [w376] -> _
                shift-left: w372 -> [w382]
                shift-right: [w377] -> w371
                shift-left: w373 -> [w379]
                tunnel: [w374] -> w370
                stop <- w375 stop-if-true
                n192 = call "CRYAPI SPLITE.vi"("nData"=w382, "sAction"="GET_SPLITER") -> ("tSpliter_Out"=w384:T4)  [unwired: 4 in, 5 out]
                n193 = Unbundle By Name(w384) -> ("nTypeP"=w381:i32, "nIDParent"=w378:i32)
                n194 = Equal To 0?(x=w381) -> (x = 0?=w380:bool)
                n195 = case shown="True" w380 {
                  tunnel: w379 -> [w388 _]
                  tunnel: w378 -> [w386 w396]
                  tunnel: [w388 w395] -> w377
                  tunnel: [FALSE w394] -> w375
                  tunnel: [w386 w393] -> w376
                  tunnel: [0 w391] -> w374
                  frame False {
                  }
                  frame True {
                    n196 = call "CRYAPI FRAME.vi"("nData"=w396, "sAction"="GET_FRAME") -> ("tFrame_Out"=w395:T2)  [unwired: 4 in, 5 out]
                    n197 = Unbundle By Name(w395) -> ("nParent"=w393:i32, "nID"=w392:i32, "nTypeF"=w390:i32, "nType"=w389:i32)
                    n198 = case shown="Default" w392 {
                      tunnel: [w398 1] -> w391
                      tunnel: w390 -> [w400 _]
                      tunnel: w389 -> [w399 _]
                      frame Default {
                        n199 = case shown="1" w400 {
                          tunnel: w399 -> [w402 w406]
                          tunnel: [w401 w405] -> w398
                          frame 0, Default {
                            n200 = case shown="0" w402 {
                              tunnel: [2 4] -> w401
                              frame 0 {
                              }
                              frame Default {
                              }
                            }
                          }
                          frame 1 {
                            n201 = case shown="Default" w406 {
                              tunnel: [3 5] -> w405
                              frame 0 {
                              }
                              frame Default {
                              }
                            }
                          }
                        }
                      }
                      frame 1 {
                      }
                    }
                    n202 = Equal To 0?(x=w393) -> (x = 0?=w394:bool)
                  }
                }
              }
            }
          }
        }
      }
      n203 = local write "nData_Out"(w350) -> ()
      n204 = local write "tFrame_Out"(w349) -> ()
    }
    frame "IS_DOCUMENT" {
      n205 = call "CRYAPI FRAME.vi"("nData"=w468, "sAction"="GET_FRAME") -> ("sData_Out"=w467:string, "tFrame_Out"=w462:T2)  [unwired: 4 in, 4 out]
      n206 = call "CRYAPI FRAME.vi"("sData"="Document" ("Window Type"), "sAction"="FIND_WIN") -> ("sData_Out"=w466:string, "tFrame_Out"=w463:T2)  [unwired: 4 in, 4 out]
      n207 = Equal?(x=w466, y="OPEN") -> (x = y?=w464:bool)
      n208 = case shown="True" w464 {
        tunnel: [0 w477] -> w471
        tunnel: w467 -> [_ w481]
        tunnel: w463 -> [_ w480]
        tunnel: w462 -> [_ w479]
        frame False {
        }
        frame True {
          n209 = case shown="\"_FRAME\"" w481 {
            tunnel: [0 w491 w495] -> w478
            tunnel: w480 -> [_ _ w498]
            tunnel: w479 -> [_ w493 w500]
            tunnel: [FALSE FALSE TRUE] -> w474
            frame Default {
            }
            frame "_TAB" {
              n210 = Unbundle By Name(w493) -> ("nID"=w491:i32)
            }
            frame "_FRAME" {
              n211 = Unbundle By Name(w498) -> ("nID"=w497:i32)
              n212 = call "CRYAPI REMOVE.vi"("tFrame"=w500, "sAction"="GET_LIST_WIN") -> ("List_ID_Out"=w499:i32[])  [unwired: 3 in, 6 out]
              n213 = for {
                tunnel: w499 -> [w506] mode=indexing
                tunnel: w497 -> [w505]
                shift-right: [w503] -> w495
                shift-left: 0 ("nData_Out") -> [w502]
                stop <- w504 stop-if-true
                n214 = Equal?(x=w506, y=w505) -> (x = y?=w504:bool)
                n215 = case shown="True" w504 {
                  tunnel: w505 -> [_ w508]
                  tunnel: [w507 w508] -> w503
                  tunnel: w502 -> [w507 _]
                  frame False {
                  }
                  frame True {
                  }
                }
              }
            }
          }
          n216 = Not Equal To 0?(x=w478) -> (x != 0?=w475:bool)
          n217 = And(x=w475, y=w474) -> (x .and. y?=w476:bool)
          n218 = case shown="True" w476 {
            tunnel: w478 -> [w482 w483]
            tunnel: [w482 w484] -> w477
            frame False {
            }
            frame True {
              n219 = call "CRYAPI FRAME.vi"("nData"=w483, "sAction"="GET_FRAME") -> ("tFrame_Out"=w487:T2)  [unwired: 4 in, 5 out]
              n220 = Unbundle By Name(w487) -> ("nParent"=w485:i32)
              n221 = Greater Than 0?(x=w485) -> (x > 0?=w486:bool)
              n222 = Select(t=w485, s=w486, f=w483) -> (s? t:f=w484:i32)
            }
          }
        }
      }
      n223 = local write "nData_Out"(w471) -> ()
    }
    frame "CLOSE_FRAME_BY_ID", "CLOSE_FRAME_BY_tFRAME" {
      # "Close One Frame"
      n224 = case shown="\"CLOSE_FRAME_BY_ID\"" w510 {
        tunnel: w512 -> [_ w524]
        tunnel: [w522 w523] -> w511
        tunnel: w509 -> [w522 _]
        frame "CLOSE_FRAME_BY_tFRAME", Default {
        }
        frame "CLOSE_FRAME_BY_ID" {
          n225 = call "CRYAPI FRAME.vi"("nData"=w524, "sAction"="GET_FRAME") -> ("tFrame_Out"=w523:T2)  [unwired: 4 in, 5 out]
        }
      }
      n226 = Unbundle By Name(w511) -> ("nParent"=w516:i32)
      n227 = case shown="Default" w516 {
        tunnel: w511 -> [w531 w532]
        tunnel: [w526 w533] -> w515
        frame 0 {
          n228 = Bundle By Name(cluster=w531, "nDockID"=0, "nDockLR"=0) -> (w527:T2)
          n229 = call "CRYAPI FRAME.vi"("tFrame"=w527, "sAction"="REPLACE_FRAME") -> ("tFrame_Out"=w526:T2)  [unwired: 4 in, 5 out]
        }
        frame Default {
          n230 = Unbundle By Name(w532) -> ("nID"=w536:i32)
          n231 = call "CRYAPI MANAGER.vi"("nData"=w536, "sAction"="FLOAT_PANEL_HIDE") -> ("nData_Out"=w537:i32)  [unwired: 3 in, 6 out]
          n232 = call "CRYAPI MANAGER.vi"("tFrame"=w532, "nData"=w537, "sAction"="FLOAT_FRAME") -> ("tFrame_Out"=w533:T2)  [unwired: 2 in, 6 out]
        }
      }
      n233 = call "CRYAPI REMOVE.vi"("tFrame"=w515, "sAction"="GET_LIST_ID") -> ("nData_Out"=w518:i32, "tFrame_Out"=w520:T2, "List_ID_Out"=w519:i32[])  [unwired: 3 in, 4 out]
      n234 = case shown="Default" w518 {
        tunnel: w519 -> [_ w541]
        tunnel: w520 -> [w538 w545]
        tunnel: [w538 w545] -> w514
        frame 0 {
        }
        frame Default {
          n235 = call "CRYAPI REMOVE.vi"("List_ID"=w541, "sAction"="GET_LIST_IDFRAME") -> ("List_ID_Out"=w546:i32[])  [unwired: 3 in, 6 out]
          n236 = call "CRYAPI REMOVE.vi"("List_ID"=w541, "sAction"="GET_LIST_IDSPLITER") -> ("List_ID_Out"=w551:i32[])  [unwired: 3 in, 6 out]
          n237 = call "CRYAPI REMOVE.vi"("List_ID"=w541, "sAction"="GET_LIST_IDWIN") -> ("List_ID_Out"=w539:i32[])  [unwired: 3 in, 6 out]
          n238 = call "CRYAPI REMOVE.vi"("List_ID"=w541, "sAction"="REMOVE_SPF") -> ("nData_Out"=w540:i32)  [unwired: 3 in, 6 out]
          n239 = call "CRYAPI REMOVE.vi"("nData"=w540, "List_ID"=w546, "sAction"="REMOVE_FRAMES") -> ("tFrame_Out"=w544:T2)  [unwired: 2 in, 6 out]
          n240 = call "CRYAPI REMOVE.vi"("nData"=w540, "tFrame"=w544, "List_ID"=w551, "sAction"="REMOVE_SPLITERS") -> ("tFrame_Out"=w543:T2)  [unwired: 1 in, 6 out]
          n241 = call "CRYAPI REMOVE.vi"("nData"=w540, "tFrame"=w543, "List_ID"=w539, "sAction"="REMOVE_FRAMES") -> ()  [unwired: 1 in, 7 out]
        }
      }
      n242 = local write "tFrame_Out"(w514) -> ()
      n243 = Unbundle By Name(w514) -> ("nID"=w513:i32)
      n244 = call "CRYAPI FRAME LIB.vi"("nData"=w513, "sAction"="REMOVE_FRAME") -> ()  [unwired: 4 in, 6 out]
    }
  }
